vi "MONITOR & WEATHER REPORT.vi"   [LabVIEW 2013]
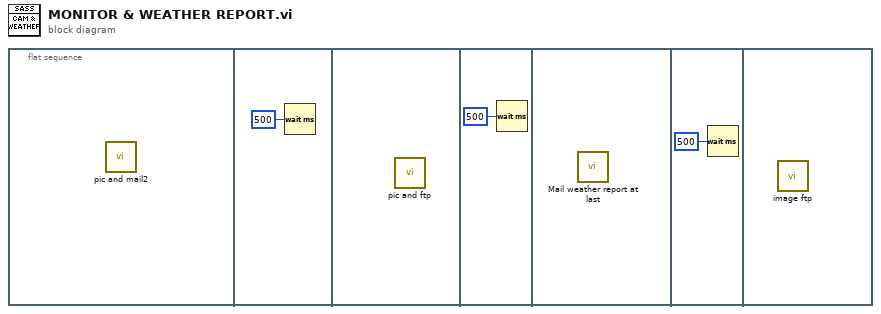
[diagram p0: block diagram]
diagram:
  n1 = flat-sequence {
    frame #0 {
      n2 = call "pic and mail2.vi"() -> ()  [unwired: 12 in]
    }
    frame #1 {
      n3 = Wait (ms)(milliseconds to wait=u32 500) -> ()  [unwired: 1 out]
    }
    frame #2 {
      n4 = call "pic and ftp.vi"() -> ()  [unwired: 12 in]
    }
    frame #3 {
      n5 = Wait (ms)(milliseconds to wait=u32 500) -> ()  [unwired: 1 out]
    }
    frame #4 {
      n6 = call "Mail weather report at last.vi"() -> ()  [unwired: 12 in]
    }
    frame #5 {
      n7 = Wait (ms)(milliseconds to wait=u32 500) -> ()  [unwired: 1 out]
    }
    frame #6 {
      n8 = call "image ftp.vi"() -> ()  [unwired: 12 in]
    }
  }
